vi "Finish.vi"   [LabVIEW 2018]
doc: "This VI is called just before exiting. It is expected to close I/O refnum, save collected data, etc."
uses:
  RefNums_DriverStation.vi
  RefNums_Actuators.vi
  RefNums_Sensors.vi
  <vilib>/Rock Robotics/WPI/Utilities/WPI_GetSetVariantRefNum.vi
types:
  T1 = typedef "WPI_RobotDriveDevRef.ctl" = cluster{"DevStatus":errorcluster, "Motors[]":T2[], "Square Inputs":bool, "Max Output":dbl}
  T2 = typedef "WPI_MotorControlDeviceRef.ctl" = cluster{"DeviceStatus":errorcluster, "Type":T3, "PWM":cluster{"PWM Channel":T4, "DeadBand":T5}, "CAN":cluster{"Device Number":u8, "SetOutput VI Ref":variant, "GetOutput VI Ref":variant, "Enable VI Ref":variant, "Disable VI Ref":variant, "Data":variant}, "Invert":bool, "DIO PWM":cluster{"PWM \"Enable\" Channel":T4, "DIOChannel":T6, "PWM Rate":dbl}}
  T3 = typedef "WPI_MotorControlType.ctl" = enum16{"PWM", "CAN", "DIO PWM"}
  T4 = typedef "FPGA_DIOPWMChannel.ctl" = enum8{"PWM 0", "PWM 1", "PWM 2", "PWM 3", "PWM 4", "PWM 5", "PWM 6", "PWM 7", "PWM 8", "PWM 9", "PWM MXP 0", "PWM MXP 1", "PWM MXP 2", "PWM MXP 3", "PWM MXP 4", "PWM MXP 5", "PWM MXP 6", "PWM MXP 7", "PWM MXP 8", "PWM MXP 9", "Invalid"}
  T5 = typedef "WPI_PWMDeadband.ctl" = cluster{"Name":string, "maxPositivePwm":i32, "minPositivePwm":i32, "centerPwm":i32, "maxNegativePwm":i32, "minNegativePwm":i32, "angularRange":u16}
  T6 = typedef "FPGA_DIOChannel.ctl" = enum8{"DIO 0", "DIO 1", "DIO 2", "DIO 3", "DIO 4", "DIO 5", "DIO 6", "DIO 7", "DIO 8", "DIO 9", "DIO MXP 0", "DIO MXP 1", "DIO MXP 2", "DIO MXP 3", "DIO MXP 4", "DIO MXP 5", "DIO MXP 6", "DIO MXP 7", "DIO MXP 8", "DIO MXP 9", "DIO MXP 10", "DIO MXP 11", "DIO MXP 12", "DIO MXP 13", "DIO MXP 14", "DIO MXP 15", "SPI Port CS1", "SPI Port CS2", "SPI Port CS3", "SPI Port MISO", "SPI Port MOSI", "Invalid"}
  T7 = typedef "WPI_AnalogChannelDevRef.ctl" = cluster{"DevStatus":errorcluster, "Analog Channel":T8}
  T8 = typedef "FPGA_AIChannel.ctl" = enum8{"AI 0", "AI 1", "AI 2", "AI 3", "AI MXP 0", "AI MXP 1", "AI MXP 2", "AI MXP 3", "Invalid"}
  T9 = typedef "WPI_ServoDeviceRef.ctl" = cluster{"DeviceStatus":errorcluster, "PWM Channel":T4, "DeadBand":T5}
  T10 = typedef "WPI_SolenoidDevRef.ctl" = cluster{"DevStatus":errorcluster, "Pneumatics Control Module":u8, "Forward Solenoid Channel":T11, "Reverse Solenoid Channel":T11}
  T11 = typedef "WPI_SolenoidChannel.ctl" = enum8{"Solenoid 0", "Solenoid 1", "Solenoid 2", "Solenoid 3", "Solenoid 4", "Solenoid 5", "Solenoid 6", "Solenoid 7", "Invalid"}
  T12 = typedef "WPI_JoystickDevRef.ctl" = cluster{"Device":T13}
  T13 = typedef "WPI_JoystickDeviceEnum.ctl" = enum16{"USB 0", "USB 1", "USB 2", "USB 3", "USB 4", "USB 5"}
  T14 = typedef "WPI_CompressorDevRef.ctl" = cluster{"DevStatus":errorcluster, "Pneumatics Control Module":u8}
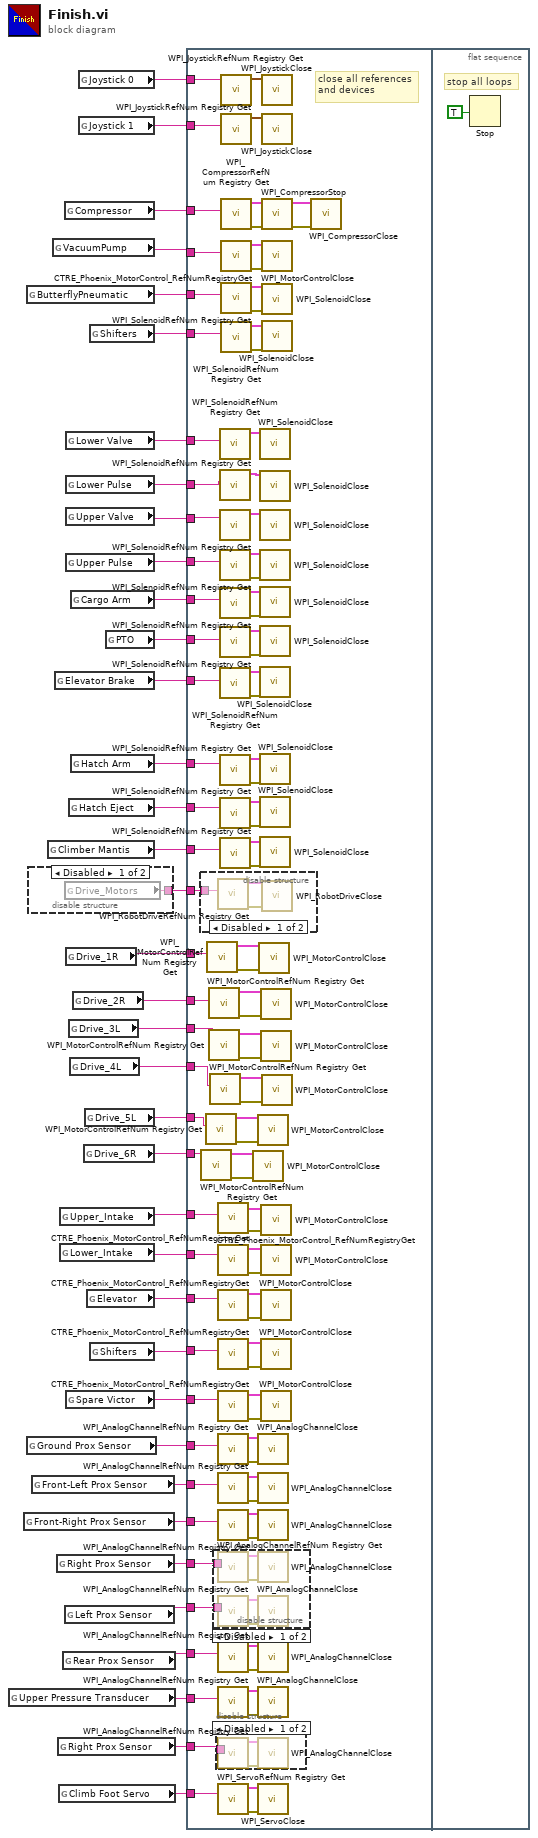
[diagram p0: block diagram]
diagram:
  n1 = global read "RefNums_Sensors.vi" "Upper Pressure Transducer"() -> (w24:string)
  n2 = global read "RefNums_Sensors.vi" "Front-Right Prox Sensor"() -> (w11:string)
  n3 = global read "RefNums_Actuators.vi" "ButterflyPneumatic"() -> (w34:string)
  n4 = global read "RefNums_Sensors.vi" "Ground Prox Sensor"() -> (w10:string)
  n5 = disable-structure shown="Disabled" {
    disable-tunnel: [w38 _] -> w8
    frame Disabled {
      n6 = global read "RefNums_Actuators.vi" "Drive_Motors"() -> (w38:string)
    }
    frame Enabled {
    }
  }
  n7 = global read "RefNums_Sensors.vi" "Front-Left Prox Sensor"() -> (w12:string)
  n8 = global read "RefNums_Actuators.vi" "Climber Mantis"() -> (w16:string)
  n9 = global read "RefNums_Actuators.vi" "VacuumPump"() -> (w32:string)
  n10 = global read "RefNums_Actuators.vi" "Elevator Brake"() -> (w19:string)
  n11 = global read "RefNums_Sensors.vi" "Right Prox Sensor"() -> (w26:string)
  n12 = global read "RefNums_Sensors.vi" "Right Prox Sensor"() -> (w9:string)
  n13 = global read "RefNums_Actuators.vi" "Climb Foot Servo"() -> (w7:string)
  n14 = global read "RefNums_Actuators.vi" "Upper_Intake"() -> (w29:string)
  n15 = global read "RefNums_Actuators.vi" "Lower_Intake"() -> (w28:string)
  n16 = global read "RefNums_Sensors.vi" "Rear Prox Sensor"() -> (w23:string)
  n17 = global read "RefNums_Actuators.vi" "Compressor"() -> (w35:string)
  n18 = global read "RefNums_Sensors.vi" "Left Prox Sensor"() -> (w25:string)
  n19 = global read "RefNums_Actuators.vi" "Lower Valve"() -> (w14:string)
  n20 = global read "RefNums_Actuators.vi" "Lower Pulse"() -> (w13:string)
  n21 = global read "RefNums_Actuators.vi" "Upper Valve"() -> (w15:string)
  n22 = global read "RefNums_Actuators.vi" "Upper Pulse"() -> (w31:string)
  n23 = global read "RefNums_Actuators.vi" "Drive_1R"() -> (w6:string)
  n24 = global read "RefNums_Actuators.vi" "Spare Victor"() -> (w21:string)
  n25 = global read "RefNums_Actuators.vi" "Hatch Eject"() -> (w17:string)
  n26 = global read "RefNums_Actuators.vi" "Drive_3L"() -> (w4:string)
  n27 = global read "RefNums_Actuators.vi" "Drive_4L"() -> (w3:string)
  n28 = global read "RefNums_Actuators.vi" "Cargo Arm"() -> (w30:string)
  n29 = global read "RefNums_Actuators.vi" "Hatch Arm"() -> (w18:string)
  n30 = global read "RefNums_Actuators.vi" "Drive_2R"() -> (w5:string)
  n31 = global read "RefNums_DriverStation.vi" "Joystick 0"() -> (w36:string)
  n32 = global read "RefNums_DriverStation.vi" "Joystick 1"() -> (w37:string)
  n33 = global read "RefNums_Actuators.vi" "Drive_6R"() -> (w1:string)
  n34 = global read "RefNums_Actuators.vi" "Drive_5L"() -> (w2:string)
  n35 = global read "RefNums_Actuators.vi" "Elevator"() -> (w27:string)
  n36 = global read "RefNums_Actuators.vi" "Shifters"() -> (w33:string)
  n37 = global read "RefNums_Actuators.vi" "Shifters"() -> (w22:string)
  n38 = global read "RefNums_Actuators.vi" "PTO"() -> (w20:string)
  n39 = flat-sequence {
    tunnel: w37 -> [w137]
    tunnel: w36 -> [w138]
    tunnel: w35 -> [w134]
    tunnel: w34 -> [w133]
    tunnel: w33 -> [w128]
    tunnel: w32 -> [w127]
    tunnel: w31 -> [w125]
    tunnel: w30 -> [w122]
    tunnel: w29 -> [w120]
    tunnel: w28 -> [w118]
    tunnel: w27 -> [w116]
    tunnel: w26 -> [w115]
    tunnel: w25 -> [w100]
    tunnel: w23 -> [w99]
    tunnel: w24 -> [w98]
    tunnel: w22 -> [w95]
    tunnel: w21 -> [w93]
    tunnel: w20 -> [w87]
    tunnel: w19 -> [w86]
    tunnel: w18 -> [w79]
    tunnel: w17 -> [w78]
    tunnel: w16 -> [w77]
    tunnel: w15 -> [w73]
    tunnel: w14 -> [w72]
    tunnel: w13 -> [w71]
    tunnel: w12 -> [w66]
    tunnel: w11 -> [w65]
    tunnel: w10 -> [w62]
    tunnel: w9 -> [w61]
    tunnel: w8 -> [w60]
    tunnel: w7 -> [w59]
    tunnel: w6 -> [w54]
    tunnel: w5 -> [w43]
    tunnel: w4 -> [w42]
    tunnel: w3 -> [w41]
    tunnel: w2 -> [w40]
    tunnel: w1 -> [w39]
    frame #0 {
      # "close all references\nand devices"
      n40 = disable-structure shown="Disabled" {
        disable-tunnel: w60 -> [w139 _]
        frame Disabled {
          n41 = call <vilib>:"WPI_RobotDriveRefNum Registry Get.vi"("refnum name"=w139) -> ("error out"=w141:errorcluster, "RobotDriveDevRef"=w140:T1)  [unwired: 9 in]
          n42 = call <vilib>:"WPI_RobotDriveClose.vi"("error in (no error)"=w141, "RobotDriveDevRef"=w140) -> ()  [unwired: 9 in, 1 out]
        }
        frame Enabled {
        }
      }
      n43 = call <vilib>:"WPI_MotorControlRefNum Registry Get.vi"("refnum name"=w39) -> ("error out"=w45:errorcluster, "MotorControlDevRef"=w44:T2)  [unwired: 9 in]
      n44 = call <vilib>:"WPI_MotorControlRefNum Registry Get.vi"("refnum name"=w40) -> ("error out"=w47:errorcluster, "MotorControlDevRef"=w46:T2)  [unwired: 9 in]
      n45 = call <vilib>:"WPI_MotorControlRefNum Registry Get.vi"("refnum name"=w54) -> ("error out"=w56:errorcluster, "MotorControlDevRef"=w55:T2)  [unwired: 9 in]
      n46 = call <vilib>:"WPI_MotorControlRefNum Registry Get.vi"("refnum name"=w43) -> ("error out"=w53:errorcluster, "MotorControlDevRef"=w52:T2)  [unwired: 9 in]
      n47 = call <vilib>:"WPI_MotorControlRefNum Registry Get.vi"("refnum name"=w42) -> ("error out"=w51:errorcluster, "MotorControlDevRef"=w50:T2)  [unwired: 9 in]
      n48 = call <vilib>:"WPI_MotorControlRefNum Registry Get.vi"("refnum name"=w41) -> ("error out"=w49:errorcluster, "MotorControlDevRef"=w48:T2)  [unwired: 9 in]
      n49 = disable-structure shown="Disabled" {
        disable-tunnel: w115 -> [w149 _]
        disable-tunnel: w100 -> [w145 _]
        frame Disabled {
          n50 = call <vilib>:"WPI_AnalogChannelRefNum Registry Get.vi"("refnum name"=w149) -> ("error out"=w148:errorcluster, "AIDeviceRef"=w150:T7)  [unwired: 9 in]
          n51 = call <vilib>:"WPI_AnalogChannelRefNum Registry Get.vi"("refnum name"=w145) -> ("error out"=w146:errorcluster, "AIDeviceRef"=w147:T7)  [unwired: 9 in]
          n52 = call <vilib>:"WPI_AnalogChannelClose.vi"("error in (no error)"=w148, "AIDeviceRef"=w150) -> ()  [unwired: 9 in, 1 out]
          n53 = call <vilib>:"WPI_AnalogChannelClose.vi"("error in (no error)"=w146, "AIDeviceRef"=w147) -> ()  [unwired: 9 in, 1 out]
        }
        frame Enabled {
        }
      }
      n54 = disable-structure shown="Disabled" {
        disable-tunnel: w61 -> [w142 _]
        frame Disabled {
          n55 = call <vilib>:"WPI_AnalogChannelRefNum Registry Get.vi"("refnum name"=w142) -> ("error out"=w144:errorcluster, "AIDeviceRef"=w143:T7)  [unwired: 9 in]
          n56 = call <vilib>:"WPI_AnalogChannelClose.vi"("error in (no error)"=w144, "AIDeviceRef"=w143) -> ()  [unwired: 9 in, 1 out]
        }
        frame Enabled {
        }
      }
      n57 = call <vilib>:"CTRE_Phoenix_MotorControl_RefNumRegistryGet.vi"("refnum name"=w120) -> ("error out"=w112:errorcluster, "PhoenixMotorControlDevRef"=w121:T2)  [unwired: 9 in]
      n58 = call <vilib>:"CTRE_Phoenix_MotorControl_RefNumRegistryGet.vi"("refnum name"=w118) -> ("error out"=w113:errorcluster, "PhoenixMotorControlDevRef"=w119:T2)  [unwired: 9 in]
      n59 = call <vilib>:"CTRE_Phoenix_MotorControl_RefNumRegistryGet.vi"("refnum name"=w116) -> ("error out"=w114:errorcluster, "PhoenixMotorControlDevRef"=w117:T2)  [unwired: 9 in]
      n60 = call <vilib>:"CTRE_Phoenix_MotorControl_RefNumRegistryGet.vi"("refnum name"=w95) -> ("error out"=w97:errorcluster, "PhoenixMotorControlDevRef"=w96:T2)  [unwired: 9 in]
      n61 = call <vilib>:"CTRE_Phoenix_MotorControl_RefNumRegistryGet.vi"("refnum name"=w93) -> ("error out"=w94:errorcluster, "PhoenixMotorControlDevRef"=w92:T2)  [unwired: 9 in]
      n62 = call <vilib>:"WPI_AnalogChannelRefNum Registry Get.vi"("refnum name"=w62) -> ("error out"=w63:errorcluster, "AIDeviceRef"=w64:T7)  [unwired: 9 in]
      n63 = call <vilib>:"WPI_AnalogChannelRefNum Registry Get.vi"("refnum name"=w66) -> ("error out"=w67:errorcluster, "AIDeviceRef"=w68:T7)  [unwired: 9 in]
      n64 = call <vilib>:"WPI_AnalogChannelRefNum Registry Get.vi"("refnum name"=w65) -> ("error out"=w69:errorcluster, "AIDeviceRef"=w70:T7)  [unwired: 9 in]
      n65 = call <vilib>:"WPI_AnalogChannelRefNum Registry Get.vi"("refnum name"=w99) -> ("error out"=w103:errorcluster, "AIDeviceRef"=w104:T7)  [unwired: 9 in]
      n66 = call <vilib>:"WPI_AnalogChannelRefNum Registry Get.vi"("refnum name"=w98) -> ("error out"=w101:errorcluster, "AIDeviceRef"=w102:T7)  [unwired: 9 in]
      n67 = call <vilib>:"WPI_ServoRefNum Registry Get.vi"("refnum name"=w59) -> ("error out"=w58:errorcluster, "ServoDeviceRef"=w57:T9)  [unwired: 9 in]
      n68 = call <vilib>:"WPI_SolenoidRefNum Registry Get.vi"("refnum name"=w72) -> ("SolenoidDevRef"=w76:T10)  [unwired: 9 in, 1 out]
      n69 = call <vilib>:"WPI_SolenoidRefNum Registry Get.vi"("refnum name"=w71) -> ("SolenoidDevRef"=w75:T10)  [unwired: 9 in, 1 out]
      n70 = call <vilib>:"WPI_SolenoidRefNum Registry Get.vi"("refnum name"=w73) -> ("SolenoidDevRef"=w74:T10)  [unwired: 9 in, 1 out]
      n71 = call <vilib>:"WPI_SolenoidRefNum Registry Get.vi"("refnum name"=w125) -> ("error out"=w110:errorcluster, "SolenoidDevRef"=w124:T10)  [unwired: 9 in]
      n72 = call <vilib>:"WPI_SolenoidRefNum Registry Get.vi"("refnum name"=w122) -> ("error out"=w111:errorcluster, "SolenoidDevRef"=w123:T10)  [unwired: 9 in]
      n73 = call <vilib>:"WPI_SolenoidRefNum Registry Get.vi"("refnum name"=w87) -> ("error out"=w90:errorcluster, "SolenoidDevRef"=w91:T10)  [unwired: 9 in]
      n74 = call <vilib>:"WPI_SolenoidRefNum Registry Get.vi"("refnum name"=w86) -> ("error out"=w88:errorcluster, "SolenoidDevRef"=w89:T10)  [unwired: 9 in]
      n75 = call <vilib>:"WPI_SolenoidRefNum Registry Get.vi"("refnum name"=w79) -> ("error out"=w84:errorcluster, "SolenoidDevRef"=w85:T10)  [unwired: 9 in]
      n76 = call <vilib>:"WPI_SolenoidRefNum Registry Get.vi"("refnum name"=w78) -> ("error out"=w82:errorcluster, "SolenoidDevRef"=w83:T10)  [unwired: 9 in]
      n77 = call <vilib>:"WPI_SolenoidRefNum Registry Get.vi"("refnum name"=w77) -> ("error out"=w80:errorcluster, "SolenoidDevRef"=w81:T10)  [unwired: 9 in]
      n78 = call <vilib>:"WPI_JoystickRefNum Registry Get.vi"("refnum name"=w138) -> ("JoystickDevRef"=w135:T12)  [unwired: 9 in, 1 out]
      n79 = call <vilib>:"WPI_JoystickRefNum Registry Get.vi"("refnum name"=w137) -> ("JoystickDevRef"=w136:T12)  [unwired: 9 in, 1 out]
      n80 = call <vilib>:"WPI_CompressorRefNum Registry Get.vi"("refnum name"=w134) -> ("error out"=w106:errorcluster, "CompressorDevRef"=w131:T14)  [unwired: 9 in]
      n81 = call <vilib>:"CTRE_Phoenix_MotorControl_RefNumRegistryGet.vi"("refnum name"=w127) -> ("error out"=w107:errorcluster, "PhoenixMotorControlDevRef"=w126:T2)  [unwired: 9 in]
      n82 = call <vilib>:"WPI_SolenoidRefNum Registry Get.vi"("refnum name"=w133) -> ("error out"=w108:errorcluster, "SolenoidDevRef"=w132:T10)  [unwired: 9 in]
      n83 = call <vilib>:"WPI_SolenoidRefNum Registry Get.vi"("refnum name"=w128) -> ("error out"=w109:errorcluster, "SolenoidDevRef"=w129:T10)  [unwired: 9 in]
      n84 = call <vilib>:"WPI_MotorControlClose.vi"("error in"=w45, "MotorControlDevRef"=w44) -> ()  [unwired: 9 in, 1 out]
      n85 = call <vilib>:"WPI_MotorControlClose.vi"("error in"=w47, "MotorControlDevRef"=w46) -> ()  [unwired: 9 in, 1 out]
      n86 = call <vilib>:"WPI_AnalogChannelClose.vi"("error in (no error)"=w63, "AIDeviceRef"=w64) -> ()  [unwired: 9 in, 1 out]
      n87 = call <vilib>:"WPI_AnalogChannelClose.vi"("error in (no error)"=w67, "AIDeviceRef"=w68) -> ()  [unwired: 9 in, 1 out]
      n88 = call <vilib>:"WPI_AnalogChannelClose.vi"("error in (no error)"=w69, "AIDeviceRef"=w70) -> ()  [unwired: 9 in, 1 out]
      n89 = call <vilib>:"WPI_AnalogChannelClose.vi"("error in (no error)"=w103, "AIDeviceRef"=w104) -> ()  [unwired: 9 in, 1 out]
      n90 = call <vilib>:"WPI_AnalogChannelClose.vi"("error in (no error)"=w101, "AIDeviceRef"=w102) -> ()  [unwired: 9 in, 1 out]
      n91 = call <vilib>:"WPI_ServoClose.vi"("error in (no error)"=w58, "ServoDeviceRef"=w57) -> ()  [unwired: 9 in, 1 out]
      n92 = call <vilib>:"WPI_MotorControlClose.vi"("error in"=w56, "MotorControlDevRef"=w55) -> ()  [unwired: 9 in, 1 out]
      n93 = call <vilib>:"WPI_SolenoidClose.vi"("SolenoidDevRef"=w76) -> ()  [unwired: 10 in, 1 out]
      n94 = call <vilib>:"WPI_SolenoidClose.vi"("SolenoidDevRef"=w75) -> ()  [unwired: 10 in, 1 out]
      n95 = call <vilib>:"WPI_SolenoidClose.vi"("SolenoidDevRef"=w74) -> ()  [unwired: 10 in, 1 out]
      n96 = call <vilib>:"WPI_SolenoidClose.vi"("error in (no error)"=w110, "SolenoidDevRef"=w124) -> ()  [unwired: 9 in, 1 out]
      n97 = call <vilib>:"WPI_SolenoidClose.vi"("error in (no error)"=w111, "SolenoidDevRef"=w123) -> ()  [unwired: 9 in, 1 out]
      n98 = call <vilib>:"WPI_SolenoidClose.vi"("error in (no error)"=w90, "SolenoidDevRef"=w91) -> ()  [unwired: 9 in, 1 out]
      n99 = call <vilib>:"WPI_SolenoidClose.vi"("error in (no error)"=w88, "SolenoidDevRef"=w89) -> ()  [unwired: 9 in, 1 out]
      n100 = call <vilib>:"WPI_SolenoidClose.vi"("error in (no error)"=w84, "SolenoidDevRef"=w85) -> ()  [unwired: 9 in, 1 out]
      n101 = call <vilib>:"WPI_SolenoidClose.vi"("error in (no error)"=w82, "SolenoidDevRef"=w83) -> ()  [unwired: 9 in, 1 out]
      n102 = call <vilib>:"WPI_SolenoidClose.vi"("error in (no error)"=w80, "SolenoidDevRef"=w81) -> ()  [unwired: 9 in, 1 out]
      n103 = call <vilib>:"WPI_MotorControlClose.vi"("error in"=w53, "MotorControlDevRef"=w52) -> ()  [unwired: 9 in, 1 out]
      n104 = call <vilib>:"WPI_MotorControlClose.vi"("error in"=w51, "MotorControlDevRef"=w50) -> ()  [unwired: 9 in, 1 out]
      n105 = call <vilib>:"WPI_MotorControlClose.vi"("error in"=w112, "MotorControlDevRef"=w121) -> ()  [unwired: 9 in, 1 out]
      n106 = call <vilib>:"WPI_MotorControlClose.vi"("error in"=w113, "MotorControlDevRef"=w119) -> ()  [unwired: 9 in, 1 out]
      n107 = call <vilib>:"WPI_MotorControlClose.vi"("error in"=w114, "MotorControlDevRef"=w117) -> ()  [unwired: 9 in, 1 out]
      n108 = call <vilib>:"WPI_MotorControlClose.vi"("error in"=w97, "MotorControlDevRef"=w96) -> ()  [unwired: 9 in, 1 out]
      n109 = call <vilib>:"WPI_MotorControlClose.vi"("error in"=w94, "MotorControlDevRef"=w92) -> ()  [unwired: 9 in, 1 out]
      n110 = call <vilib>:"WPI_JoystickClose.vi"("JoystickDevRef"=w135) -> ()  [unwired: 11 in]
      n111 = call <vilib>:"WPI_JoystickClose.vi"("JoystickDevRef"=w136) -> ()  [unwired: 11 in]
      n112 = call <vilib>:"WPI_CompressorStop.vi"("error in (no error)"=w106, "CompressorDevRef"=w131) -> ("error out"=w105:errorcluster, "CompressorDevRef"=w130:T14)  [unwired: 8 in]
      n113 = call <vilib>:"WPI_MotorControlClose.vi"("error in"=w107, "MotorControlDevRef"=w126) -> ()  [unwired: 9 in, 1 out]
      n114 = call <vilib>:"WPI_SolenoidClose.vi"("error in (no error)"=w108, "SolenoidDevRef"=w132) -> ()  [unwired: 9 in, 1 out]
      n115 = call <vilib>:"WPI_SolenoidClose.vi"("error in (no error)"=w109, "SolenoidDevRef"=w129) -> ()  [unwired: 9 in, 1 out]
      n116 = call <vilib>:"WPI_MotorControlClose.vi"("error in"=w49, "MotorControlDevRef"=w48) -> ()  [unwired: 9 in, 1 out]
      n117 = call <vilib>:"WPI_CompressorClose.vi"("error in (no error)"=w105, "CompressorDevRef"=w130) -> ()  [unwired: 9 in, 1 out]
    }
    frame #1 {
      # "stop all loops"
      n118 = Stop(stop? (T)=TRUE ("Quit")) -> ()
    }
  }
